vi "Update Color Pair Array.vi"(8 "error in (no error)":errorcluster, 9 "Color Pair Array":cluster{"Color":u32, "String":string}[](array[cluster]), 11 "3D Pie.lvclass in":refnum<class "3D Bar.lvclass">) -> (0 "error out":errorcluster, 3 "3D Pie.lvclass out":refnum<class "3D Bar.lvclass">)   [LabVIEW 2020, in "3D Bar.lvclass"]
uses:
  <vilib>/Math Plots/3D Math Plots/3D Bar/3D Bar/3D Bar.lvclass
  e:/builds/penguin/labview/branches/2020/dev/dist/vi.lib/Math Plots/3D Math Plots/3D Plot/3D Plot/3D Plot.lvclass
  <vilib>/Math Plots/3D Math Plots/3D Bar/3D Bar/3D Bar.lvclass/3D Bar.ctl
  <vilib>/Math Plots/3D Math Plots/3D Plot/3D Plot/3D Plot.lvclass
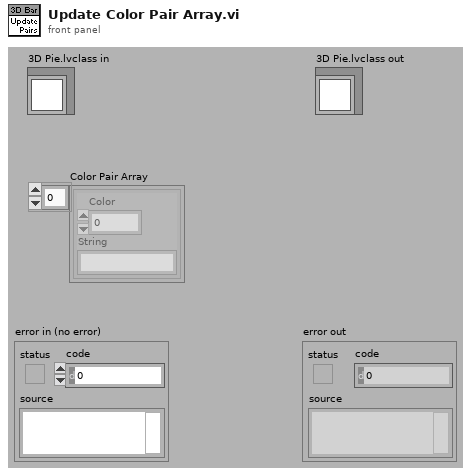
[diagram p1: front panel]
types:
  T1 = typedef "3D Bar.lvclass/3D Bar Property Array.ctl" = T2[]
  T2 = typedef "3D Bar.lvclass/3D Bar Property.ctl" = cluster{"General Property":cluster{"Plot Name":string, "Coordinate System":enum16{"Cartesian", "Cylindrical", "Spherical"}, "Opacity":sgl}, "Projection Property":cluster{"Draw XY":bool, "Draw YZ":bool, "Draw XZ":bool}, "Plot Property":cluster{"Line Style":T3, "Line Width":sgl, "Line Color":u32, "Antialiasing":bool}, "Bar Property":cluster{"Bar Mode":enum16{"Detach", "Group", "Stack"}, "Bar Width":sgl, "Color Pair Array":cluster{"Color":u32, "String":string}[]}}
  T3 = typedef "3D Plot.lvclass/Line Type.ctl" = enum16{"None", "Solid", "Dash", "Dot", "Dash Dot"}
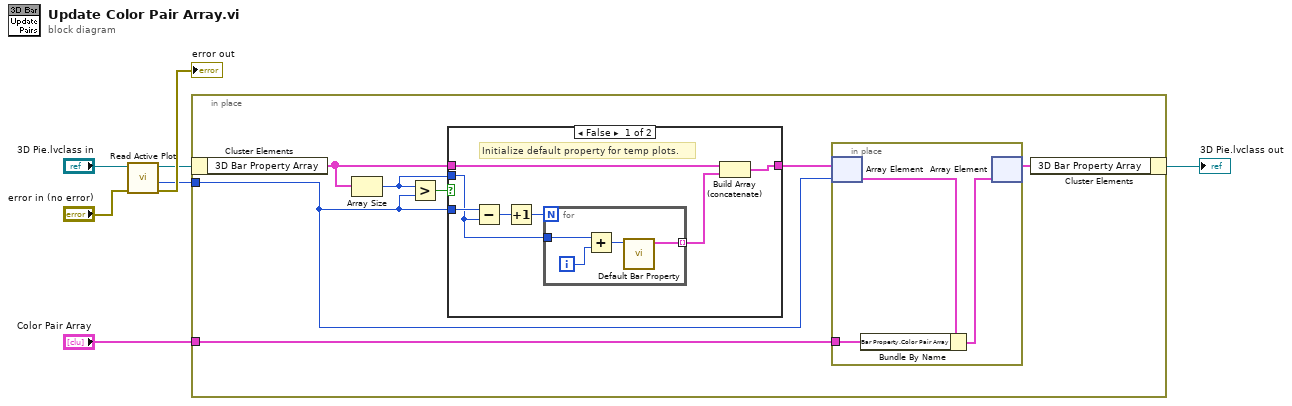
[diagram p0: block diagram]
diagram:
  n1 = call <vilib>:"Read Active Plot.vi"("error in (no error)"="error in (no error)", "3D Plot.lvclass in"="3D Pie.lvclass in") -> ("error out"=→"error out":errorcluster, "Active Plot"=w1:i32, "3D Plot.lvclass out"=w2:refnum<class "3D Bar.lvclass">)  [unwired: 7 out]
  n2 = in-place {
    in-place-border: w1 -> [w9]
    in-place-border: "Color Pair Array" -> [w10]
    n3 = in-place-cluster #1(w2) -> ("3D Bar Property Array"=w12:T1)
    n4 = Array Size(array=w12) -> (size(s)=w8:i32)
    n5 = Greater?(x=w8, y=w9) -> (0:w13:bool)
    n6 = case shown="False" w13 {
      tunnel: [w19 w26] -> w11
      tunnel: w12 -> [w21 w26]
      tunnel: w8 -> [w15 _]
      tunnel: w9 -> [w16 _]
      frame False {
        # "Initialize default property for temp plots."
        n7 = Subtract(x=w16, y=w15) -> (x-y=w18:i32)
        n8 = Increment(x=w18) -> (x+1=w17:i32)
        n9 = for {
          N: w17 -> [_]
          tunnel: w15 -> [w24]
          tunnel: [w22] -> w20 mode=indexing
          i -> [w25]
          n10 = Add(x=w24, y=w25) -> (x+y=w23:i32)
          n11 = call <vilib>:"Default Bar Property.vi"("Plot ID"=w23) -> ("Default Property"=w22:T2)  [unwired: 10 in]
        }
        n12 = Build Array (concatenate)(w21, w20) -> (w19:T1)
      }
      frame True {
      }
    }
    n13 = in-place {
      in-place-border: w10 -> [w28]
      n14 = in-place-array #2(w11, w9) -> (w29:T2)
      n15 = Bundle By Name(cluster=w29, "Bar Property.Color Pair Array"=w28) -> (w27:T2)
      n16 = in-place-array #2(w27) -> (w14:T1)  [unwired: 1 out]
    }
    n17 = in-place-cluster #1("3D Bar Property Array"=w14) -> (→"3D Pie.lvclass out":refnum<class "3D Bar.lvclass">)
  }
